vi "IDN.vi"(8 "error in (no error)":errorcluster, 11 "RP Instrument in":refnum<class "RP Instrument.lvclass">) -> (0 "error out":errorcluster, 1 "Logic tag":u16, 2 "IDN response":u32=1 format="0x%x (%d)", 3 "RP Instrument out":refnum<class "RP Instrument.lvclass">)   [LabVIEW 2016, in "RP Instrument.lvclass"]
uses:
  RP Instrument.lvclass
  RP Instrument.lvclass/RP Instrument.ctl
  RP Communicator/RP Communicator.lvclass
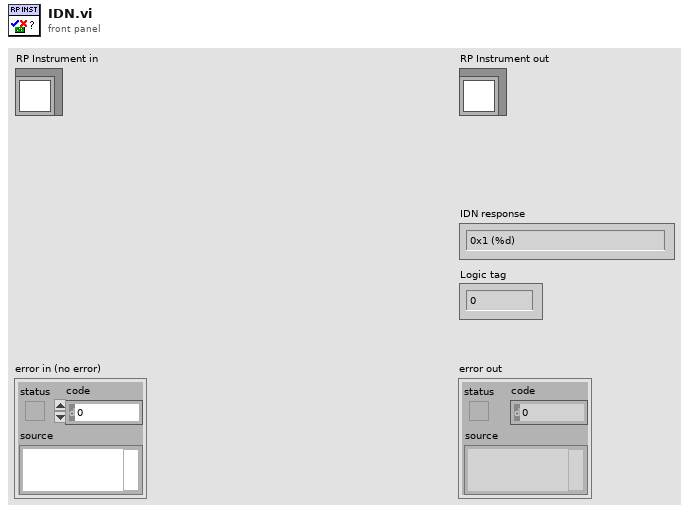
[diagram p1: front panel]
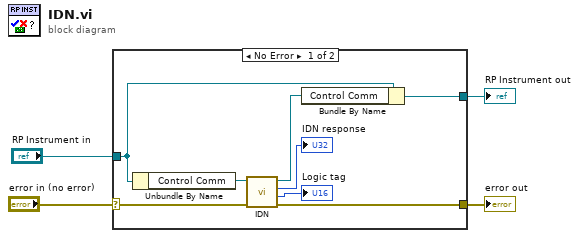
[diagram p0: block diagram]
diagram:
  n1 = case shown="No Error" "error in (no error)" {
    selector: "error in (no error)" -> [w8 w14]
    tunnel: [w7 w14] -> w3
    tunnel: [w10 w13] -> w1
    tunnel: "RP Instrument in" -> [w12 w13]
    frame No Error {
      n2 = Unbundle By Name(w12) -> ("Control Comm"=w11:refnum<class "RP Communicator.lvclass">)
      n3 = call-dynamic "IDN.vi"("error in (no error)"=w8, "RP Communicator in"=w11) -> ("error out"=w7:errorcluster, "Logic tag"=→"Logic tag":u16, "IDN response"=→"IDN response":u32, "RP Communicator out"=w9:refnum<class "RP Communicator.lvclass">)  [unwired: 6 in]
      n4 = Bundle By Name(cluster=w12, "Control Comm"=w9) -> (w10:refnum<class "RP Instrument.lvclass">)
    }
    frame Error {
    }
  }
  "error out" <- w3
  "RP Instrument out" <- w1
